vi "Pump Configure Hardware.vi"(8 "error in (no error)":errorcluster, 10 "DMM":refnum<queue>, 11 "Hardware Resources in":T1 {"Pump Info"."Direction" items=["CW", "CCW"]; "Pump Info"."Speed" format="%03.0f"}) -> (0 "error out":errorcluster, 3 "Hardware Resources out":T1 {"Pump Info"."Direction" items=["CW", "CCW"]; "Pump Info"."Speed" format="%03.0f"})   [LabVIEW 2020, in "Pump.lvlib"]
doc: "Configure the hardware."
uses:
  Pump.lvlib
  Pump Hardware Configuration.ctl
  support/Message Queue/Message Cluster.ctl
  <instrlib>/WM Pump/WM Pump.lvlib
  support/Message Queue/Message Queue.lvlib
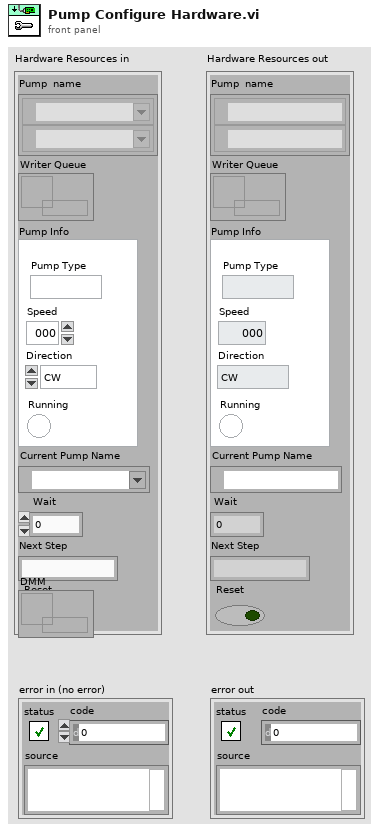
[diagram p1: front panel]
types:
  T1 = typedef "Pump.lvlib/Pump Hardware Configuration.ctl" = cluster{"Pump  name":refnum<visa-resource-name>[], "Writer Queue":refnum<queue>, "Pump Info":cluster{"Pump Type":string, "Speed":i32, "Direction":u16, "Running":bool}, "Current Pump Name":refnum<visa-resource-name>, "Wait":dbl, "Next Step":string, "Reset":bool}
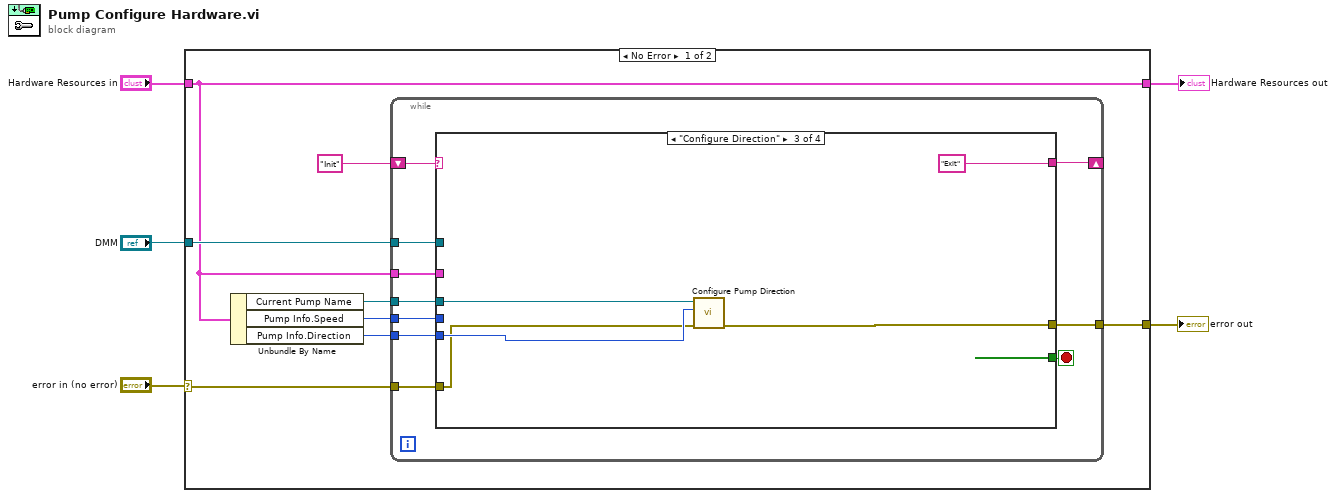
[diagram p0: block diagram]
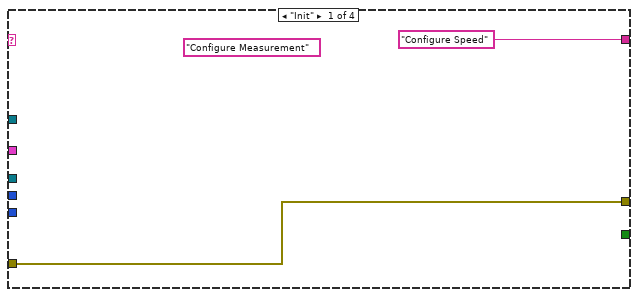
[diagram p2: hidden frame]
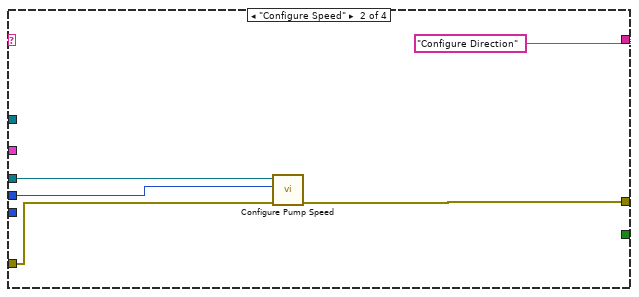
[diagram p3: hidden frame]
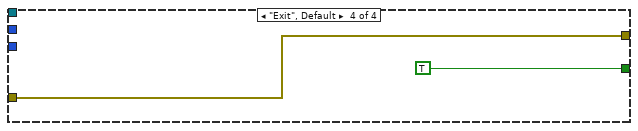
[diagram p4: hidden frame]
diagram:
  n1 = case shown="No Error" "error in (no error)" {
    selector: "error in (no error)" -> [w11 w37]
    tunnel: "DMM" -> [w12 _]
    tunnel: "Hardware Resources in" -> [w8 w36]
    tunnel: [w9 w37] -> w2
    tunnel: [w8 w36] -> w1
    frame No Error {
      n2 = Unbundle By Name(w8) -> ("Current Pump Name"=w10:refnum<visa-resource-name>, "Pump Info.Speed"=w7:i32, "Pump Info.Direction"=w6:u16)
      n3 = while {
        shift-right: [w22] -> _
        shift-left: "Init" -> [w23]
        tunnel: w12 -> [w21]
        tunnel: w11 -> [w20]
        tunnel: w10 -> [w19]
        tunnel: [w17] -> w9
        tunnel: w8 -> [w16]
        tunnel: w7 -> [w15]
        tunnel: w6 -> [w14]
        stop <- w18 stop-if-true
        n4 = case shown="\"Configure Direction\"" w23 {
          tunnel: ["Configure Speed" "Configure Direction" "Exit" _] -> w22
          tunnel: w21 -> [_ _ _ _]
          tunnel: w20 -> [w25 w28 w30 w34]
          tunnel: w19 -> [_ w27 w32 _]
          tunnel: [_ _ _ TRUE] -> w18
          tunnel: [w25 w28 w30 w34] -> w17
          tunnel: w16 -> [_ _ _ _]
          tunnel: w15 -> [_ w26 _ _]
          tunnel: w14 -> [_ _ w31 _]
          frame "Init" {
            (unwired) "Configure Measurement"
          }
          frame "Configure Speed" {
            n5 = call <instrlib>:"Configure Pump Speed.vi"("Speed"=w26, "VISA resource name"=w27) -> ()  [unwired: 8 in, 2 out]
          }
          frame "Configure Direction" {
            n6 = call <instrlib>:"Configure Pump Direction.vi"("error in (no error)"=w30, "Direction"=w31, "VISA resource name"=w32) -> ()  [unwired: 7 in, 2 out]
          }
          frame "Exit", Default {
          }
        }
      }
    }
    frame Error {
    }
  }
  "Hardware Resources out" <- w1
  "error out" <- w2
